vi "Inject Attribute List.vi"(6 "Attributes Ref":refnum<data-value>, 8 "error in (no error)":errorcluster, 11 "Stop Bug Remover in":refnum<class "Stop Air Dry.lvclass">) -> (0 "error out":errorcluster, 3 "Stop Bug Remover out":refnum<class "Stop Air Dry.lvclass">)   [LabVIEW 2019, in "Stop Air Dry.lvclass"]
uses:
  <vilib>/gpm_packages/@cs/Car-wash/Source/Process Steps/Stop Air Dry/Stop Air Dry.lvclass
  <vilib>/gpm_packages/@cs/lookup-table/Source/LookupTable/LookupTable.lvclass
  <vilib>/gpm_packages/@cs/lookup-table/Source/LookupTable/LookupTable.lvclass/LookupTable.ctl
  <vilib>/gpm_packages/@cs/Car-wash/Source/Process Steps/Stop Air Dry/Stop Air Dry.lvclass/Stop Air Dry.ctl
  f4cc7fe8-c12d-45be-8522-a993f07a4f77.vi
  <vilib>/gpm_packages/@cs/lookup-table/Source/LookupTable/Read Table Reference.vi
  f4cc7fe8-c12d-45be-8522-a993f07a4f77.vi/1efed656-9cd4-4308-a2d3-a85bd2f88506.vi
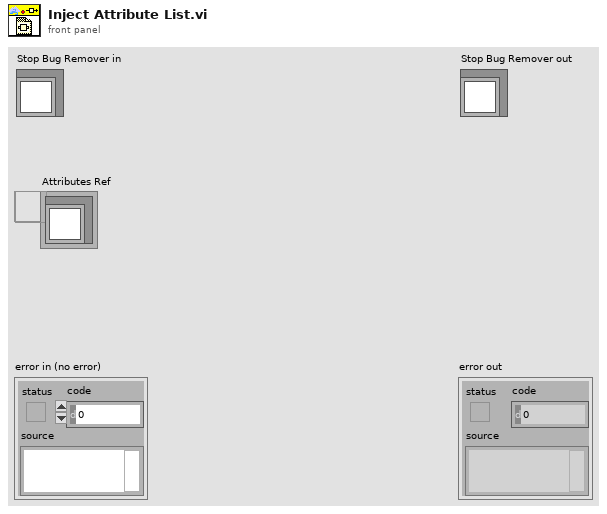
[diagram p1: front panel]
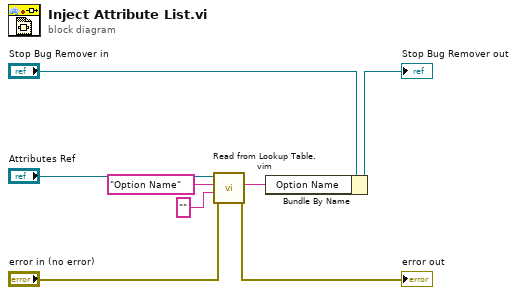
[diagram p0: block diagram]
diagram:
  n1 = call "Read from Lookup Table.vim"("error in (no error)"="error in (no error)", "Type"="", "Item Name"="Option Name", "LookupTable Reference"="Attributes Ref") -> ("error out"=→"error out":errorcluster, "Value"=w6:string)  [unwired: 4 in, 2 out]
  n2 = Bundle By Name(cluster="Stop Bug Remover in", "Option Name"=w6) -> (→"Stop Bug Remover out":refnum<class "Stop Air Dry.lvclass">)
